vi "Get Valid Data from string.vi"(11 "after substring":string) -> (3 "F-format string":string)   [LabVIEW 2021]
doc: "get valid data from string."
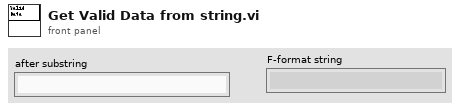
[diagram p1: front panel]
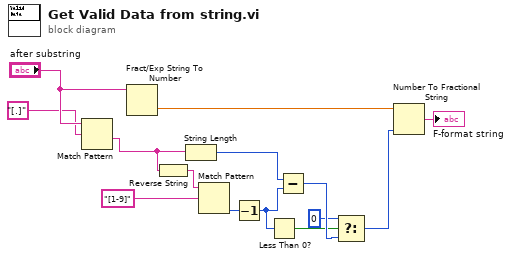
[diagram p0: block diagram]
diagram:
  n1 = Match Pattern(string="after substring", regular expression="[.]") -> (after substring=w3:string)  [unwired: 1 in, 3 out]
  n2 = Fract/Exp String To Number(string="after substring") -> (number=w12:dbl)  [unwired: 3 in, 1 out]
  n3 = Reverse String(1:w3) -> (0:w5:string)
  n4 = String Length(string=w3) -> (length=w6:i32)
  n5 = Match Pattern(string=w5, regular expression="[1-9]") -> (offset past match=w7:i32)  [unwired: 1 in, 3 out]
  n6 = Decrement(x=w7) -> (x-1=w8:i32)
  n7 = Less Than 0?(x=w8) -> (x < 0?=w10:bool)
  n8 = Subtract(x=w6, y=w8) -> (x-y=w11:i32)
  n9 = Select(t=0, s=w10, f=w11) -> (s? t:f=w2:i32)
  n10 = Number To Fractional String(number=w12, precision (6)=w2) -> (F-format string=→"F-format string":string)  [unwired: 2 in]
